vi "Get U32.vi"(8 "error in (no error)":errorcluster, 9 "Data Type (default value)":u32, 10 "Offset":i32, 11 "JSON":string) -> (0 "error out":errorcluster, 1 "Number":u32, 2 "Offset past match":i32)   [LabVIEW 2017, in "JSONtext.lvlib"]
uses:
  JSONtext.lvlib
  String Subset.vi
  Parsing/Advance past Number.vi
  support/Format Error.vi
  <vilib>/Utility/error.llb/Error Cluster From Error Code.vi
  Parsing/Parsing Error.vi
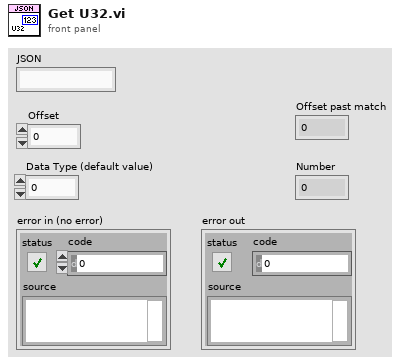
[diagram p1: front panel]
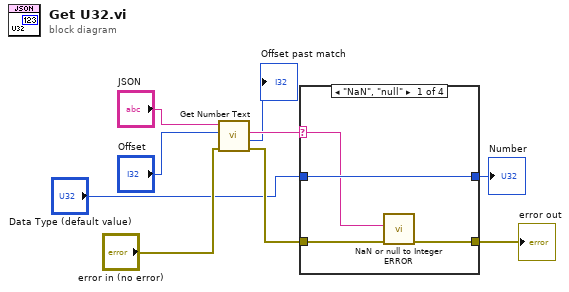
[diagram p0: block diagram]
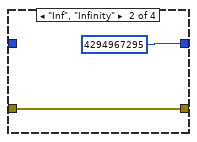
[diagram p2: hidden frame]
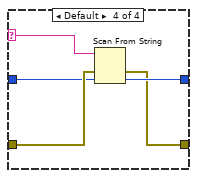
[diagram p4: hidden frame]
diagram:
  n1 = call "Get Number Text.vi"("error in (no error)"="error in (no error)", "Offset"="Offset", "JSON"="JSON") -> ("error out"=w6:errorcluster, "Offset past match"=→"Offset past match":i32, "Number Text"=w4:string)  [unwired: 5 in, 1 out]
  n2 = case shown="\"NaN\", \"null\"" w4 {
    selector: w4 -> [w10 _ _ w18]
    tunnel: [w13 u32 4294967295 ("default value 1") w16 w22] -> w3
    tunnel: w6 -> [w12 w14 w17 w21]
    tunnel: [w11 w14 w17 w20] -> w5
    tunnel: "Data Type (default value)" -> [w13 _ w16 w19]
    frame "NaN", "null" {
      n3 = call "NaN or null to Integer ERROR.vi"("error in (no error)"=w12, "JSON NaN or null"=w10) -> ("error out"=w11:errorcluster)  [unwired: 9 in]
    }
    frame "Inf", "Infinity" {
    }
    frame "-Inf", "-Infinity" {
    }
    frame Default {
      n4 = Scan From String(input string=w18, error in=w21, default 1=w19) -> (error out=w20:errorcluster, output 1=w22:u32)  [unwired: 2 in, 2 out]
    }
  }
  "error out" <- w5
  "Number" <- w3
